vi "LoadGlobais2.vi"(8 "error in (no error)":errorcluster, 10 "Mecanismo":string, 11 "Controlador in":refnum<class "Controlador.lvclass">) -> (0 "error out":errorcluster, 2 "Resp":string, 3 "Controlador out":refnum<class "Controlador.lvclass">)   [LabVIEW 2018, in "Controlador.lvclass"]
uses:
  Controlador.lvclass
  Global Coude.vi
  <vilib>/Utility/config.llb/NI_LVConfig.lvlib
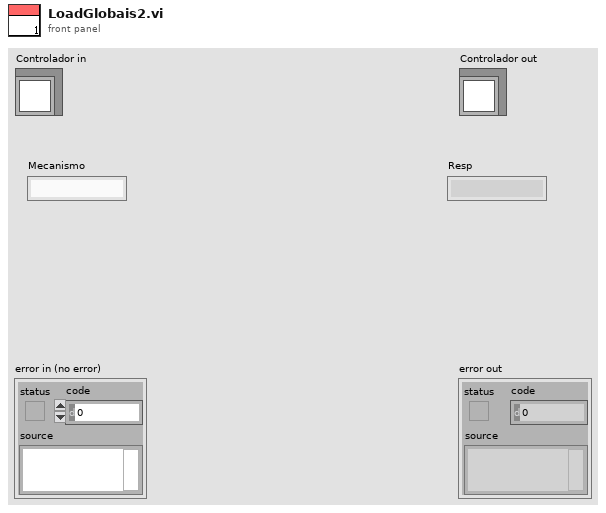
[diagram p1: front panel]
types:
  T1 = cluster{"Mec ID":string, "VISA Mec":refnum<visa-resource-name>, "Mec PosLimit":string, "Mec NegLimit":string, "MecOffset":string, "MecTargets":dbl[], "MecEnabled":bool, "Mec Target":dbl}
  T2 = typedef "NI_LVConfig.lvlib/Config Data RefNum.ctl" = refnum<k1>
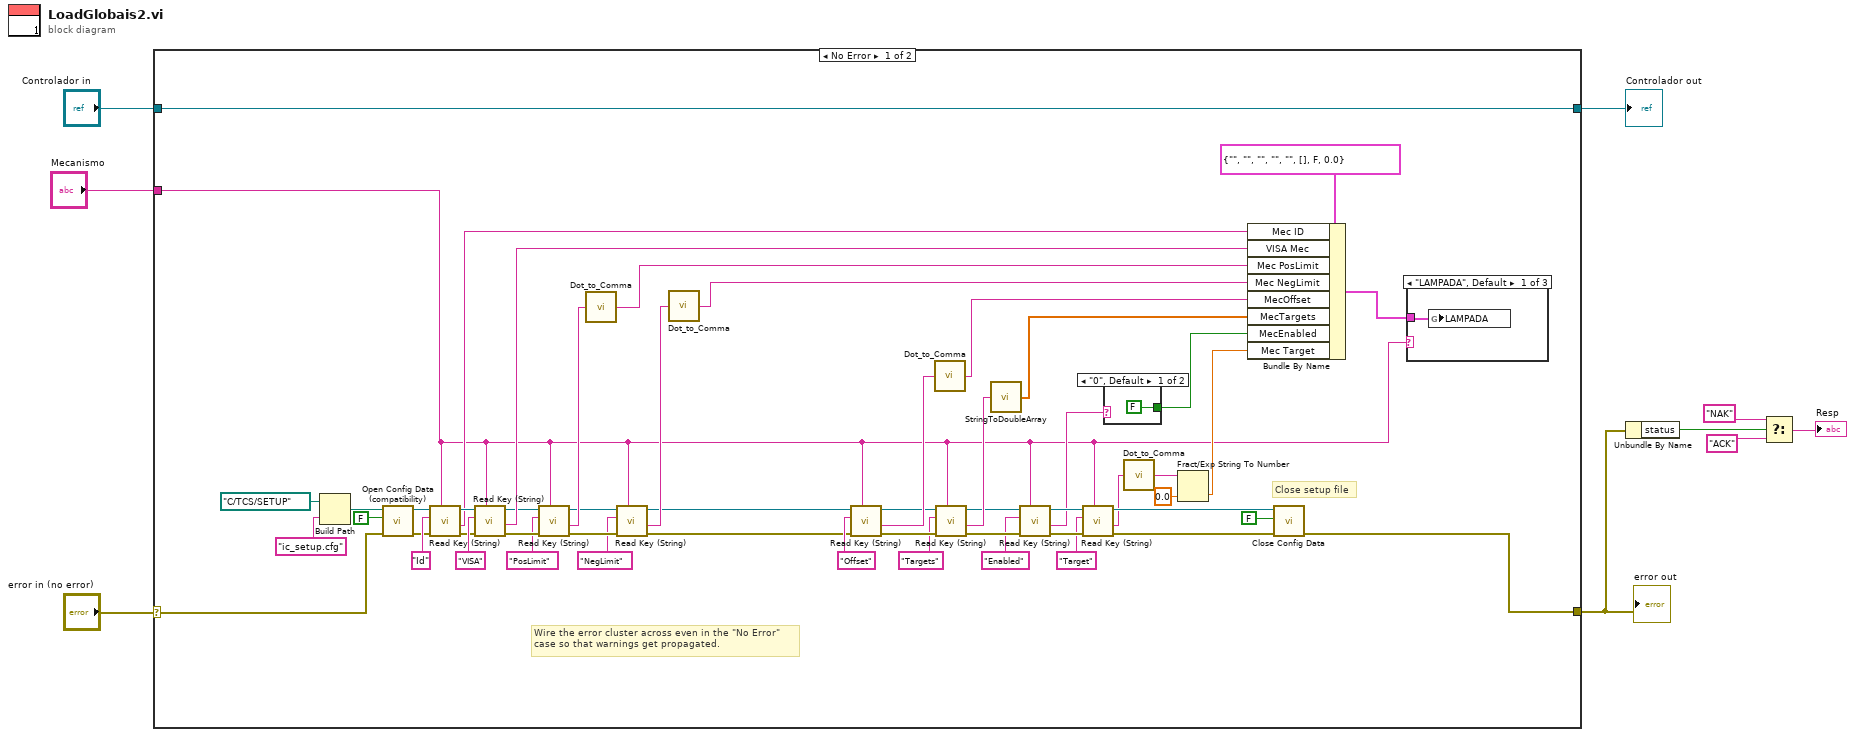
[diagram p0: block diagram]
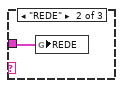
[diagram p2: hidden frame]
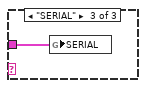
[diagram p3: hidden frame]
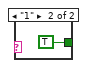
[diagram p4: hidden frame]
diagram:
  n1 = case shown="No Error" "error in (no error)" {
    selector: "error in (no error)" -> [w17 w69]
    tunnel: [w16 w69] -> w2
    tunnel: [w13 w68] -> w7
    tunnel: "Controlador in" -> [w13 w68]
    tunnel: "Mecanismo" -> [w10 _]
    frame No Error {
      # "Close setup file"
      # "Wire the error cluster across even in the \"No Error\"\ncase so that warnings get propagated."
      n2 = Build Path(base path=path "C:/TCS/SETUP", name or relative path="ic_setup.cfg") -> (appended path=w22:path)
      n3 = call <vilib>:"Open Config Data (compatibility).vi"("error in (no error)"=w17, "create file if necessary (T)"=FALSE ("create file if necessary? (T)"), "configuration file path"=w22) -> ("error out"=w20:errorcluster, "refnum"=w19:T2)  [unwired: 6 in, 1 out]
      n4 = call <vilib>:"Read Key (String).vi"("section"=w10, "error in (no error)"=w20, "key"="Id", "refnum"=w19) -> ("error out"=w24:errorcluster, "value"=w23:string, "refnum out"=w25:T2)  [unwired: 2 in, 3 out]
      n5 = call <vilib>:"Read Key (String).vi"("section"=w10, "error in (no error)"=w24, "key"="VISA", "refnum"=w25) -> ("error out"=w50:errorcluster, "value"=w58:string, "refnum out"=w49:T2)  [unwired: 2 in, 3 out]
      n6 = call <vilib>:"Read Key (String).vi"("section"=w10, "error in (no error)"=w50, "key"="PosLimit", "refnum"=w49) -> ("error out"=w52:errorcluster, "value"=w54:string, "refnum out"=w51:T2)  [unwired: 2 in, 3 out]
      n7 = call "Dot_to_Comma.vi"("String in"=w54) -> ("String out"=w59:string)
      n8 = call <vilib>:"Read Key (String).vi"("section"=w10, "error in (no error)"=w52, "key"="NegLimit", "refnum"=w51) -> ("error out"=w15:errorcluster, "value"=w55:string, "refnum out"=w14:T2)  [unwired: 2 in, 3 out]
      n9 = call "Dot_to_Comma.vi"("String in"=w55) -> ("String out"=w60:string)
      n10 = call <vilib>:"Read Key (String).vi"("section"=w10, "error in (no error)"=w15, "key"="Offset", "refnum"=w14) -> ("error out"=w46:errorcluster, "value"=w56:string, "refnum out"=w45:T2)  [unwired: 2 in, 3 out]
      n11 = call "Dot_to_Comma.vi"("String in"=w56) -> ("String out"=w61:string)
      n12 = call <vilib>:"Read Key (String).vi"("section"=w10, "error in (no error)"=w46, "key"="Targets", "refnum"=w45) -> ("error out"=w37:errorcluster, "value"=w42:string, "refnum out"=w40:T2)  [unwired: 2 in, 3 out]
      n13 = call "StringToDoubleArray.vi"("String"=w42) -> ("MecTargets"=w62:dbl[])
      n14 = call <vilib>:"Read Key (String).vi"("section"=w10, "error in (no error)"=w37, "key"="Enabled", "refnum"=w40) -> ("error out"=w36:errorcluster, "value"=w32:string, "refnum out"=w39:T2)  [unwired: 2 in, 3 out]
      n15 = call <vilib>:"Read Key (String).vi"("section"=w10, "error in (no error)"=w36, "key"="Target", "refnum"=w39) -> ("error out"=w35:errorcluster, "value"=w28:string, "refnum out"=w38:T2)  [unwired: 2 in, 3 out]
      n16 = case shown="\"0\", Default" w32 {
        tunnel: [FALSE TRUE] -> w31
        frame "0", Default {
        }
        frame "1" {
        }
      }
      n17 = call "Dot_to_Comma.vi"("String in"=w28) -> ("String out"=w30:string)
      n18 = Fract/Exp String To Number(string=w30, default (0 dbl)=0.0) -> (number=w27:dbl)  [unwired: 3 out]
      n19 = Bundle By Name(cluster=T1 {"Mec ID"="", "VISA Mec"="", "Mec PosLimit"="", "Mec NegLimit"="", "MecOffset"="", "MecTargets"=[], "MecEnabled"=FALSE, "Mec Target"=0.0} ("LAMPADA"), "Mec ID"=w23, "VISA Mec"=w58, "Mec PosLimit"=w59, "Mec NegLimit"=w60, "MecOffset"=w61, "MecTargets"=w62, "MecEnabled"=w31, "Mec Target"=w27) -> (w18:T1)
      n20 = call <vilib>:"Close Config Data.vi"("error in (no error)"=w35, "write file if changed (T)"=FALSE ("create file if necessary? (T)"), "refnum"=w38) -> ("error out"=w16:errorcluster)  [unwired: 8 out]
      n21 = case shown="\"LAMPADA\", Default" w10 {
        tunnel: w18 -> [w63 w64 w65]
        frame "LAMPADA", Default {
          n22 = global write "Global Coude.vi" "LAMPADA"(w63) -> ()
        }
        frame "REDE" {
          n23 = global write "Global Coude.vi" "REDE"(w64) -> ()
        }
        frame "SERIAL" {
          n24 = global write "Global Coude.vi" "SERIAL"(w65) -> ()
        }
      }
    }
    frame Error {
    }
  }
  "error out" <- w2
  "Controlador out" <- w7
  n25 = Unbundle By Name(w2) -> ("status"=w6:bool)
  n26 = Select(t="NAK", s=w6, f="ACK") -> (s? t:f=→"Resp":string)
